vi "CC FITS Read Image.vi"(8 "error in (no error)":errorcluster, 11 "FITS File Path":path) -> (0 "error out":errorcluster, 3 "Image":sgl[][](graph))   [LabVIEW 2024]
uses:
  gfitsio/gfitsio-read-image-subset-sgl-2d.vi
  gfitsio/gfitsio.lvlib
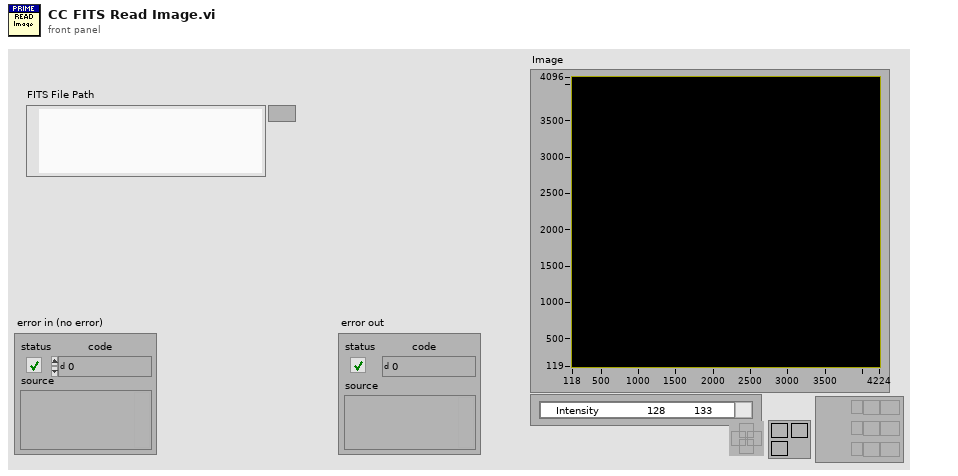
[diagram p1: front panel]
types:
  T1 = typedef "gfitsio.lvlib/gfitsio-refnum.ctl" = u64
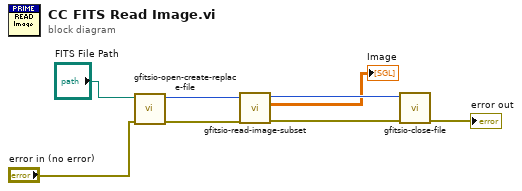
[diagram p0: block diagram]
diagram:
  n1 = call "gfitsio-open-create-replace-file.vi"("error in (no error)"="error in (no error)", "file path (dialog if empty)"="FITS File Path") -> ("error out"=w5:errorcluster, "gfits refnum"=w8:T1)  [unwired: 7 in, 1 out]
  n2 = call-poly "gfitsio-read-image-subset.vi"("error in (no error)"=w5, "gfits refnum"=w8) -> ("error out"=w4:errorcluster, "data"=→"Image":sgl[][], "dup gfits refnum"=w3:T1)  [unwired: 7 in]
  n3 = call "gfitsio-close-file.vi"("error in (no error)"=w4, "gfits refnum"=w3) -> ("error out"=→"error out":errorcluster)  [unwired: 8 in, 1 out]
